vi "Experimental Triangle Right Half Ramp.vi"() -> (0 "Left Half Triangle":waveform(dbl))   [LabVIEW 2013]
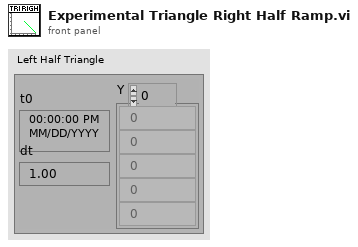
[diagram p1: front panel]
types:
  T1 = typedef "Actuation Mode.ctl" = enum16{"Up Mode", "Down Mode"}
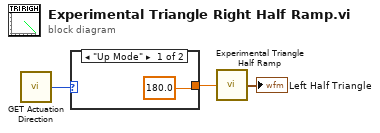
[diagram p0: block diagram]
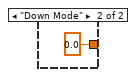
[diagram p2: hidden frame]
diagram:
  n1 = call "GET Actuation Direction.vi"() -> ("Actuation Mode"=w2:T1)
  n2 = case shown="\"Up Mode\"" w2 {
    tunnel: [180.0 0.0] -> w1
    frame "Up Mode" {
    }
    frame "Down Mode" {
    }
  }
  n3 = call "Experimental Triangle Half Ramp.vi"("Phase Offset"=w1) -> ("Half Triangle"=→"Left Half Triangle":waveform(dbl))
